vi "qDRL.vi"(0 "System no.":i32=1 min=1 max=4 step=1, 2 "Rec. table to query":i32[](array[numeric]), 3 "With Rec. table IDs?":bool, 5 "error in":errorcluster) -> (16 "No. of rec. values":i32[](array[numeric]), 19 "error out":errorcluster)   [LabVIEW 2020]
doc: "This VI returns the number of recorded data values for the given record tables. \n\nC-887, F-206, M-8X0: Only for GCS syntax version = GCS 2.0 or higher (Check with CSV?.vi. If CSV?.vi is not supported, syntax version is GCS 1.0)."
panel:
  # "Returns the number of recorded data values for the given record tables"
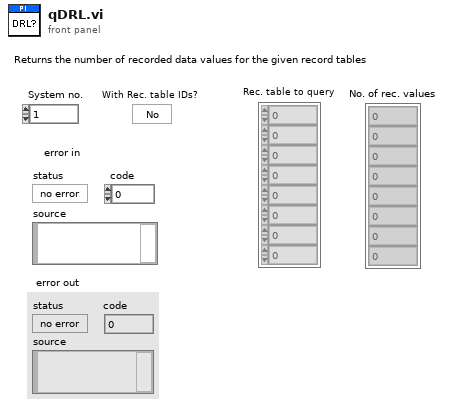
[diagram p1: front panel]
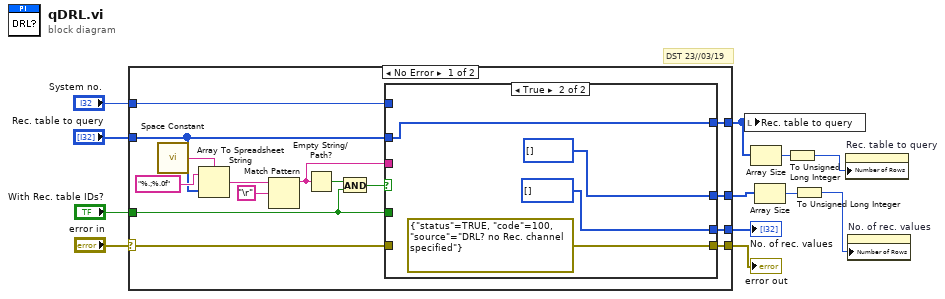
[diagram p0: block diagram]
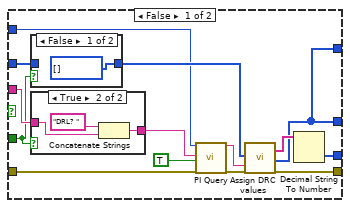
[diagram p2: hidden frame]
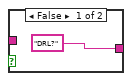
[diagram p4: hidden frame]
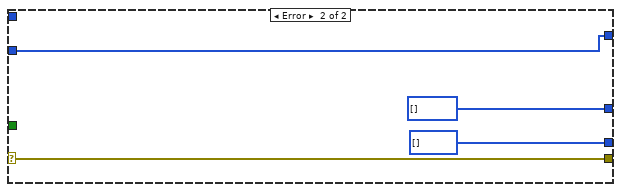
[diagram p5: hidden frame]
diagram:
  # "DST 23//03/19"
  n1 = case shown="No Error" "error in" {
    selector: "error in" -> [w17 w53]
    tunnel: "Rec. table to query" -> [w21 w52]
    tunnel: "System no." -> [w26 _]
    tunnel: [w27 w53] -> w10
    tunnel: "With Rec. table IDs?" -> [w18 _]
    tunnel: [w19 i32[] [] ("Trigger option")] -> w8
    tunnel: [w16 i32[] [] ("Queried Rec. table out")] -> w6
    tunnel: [w13 w52] -> w3
    frame No Error {
      n2 = call <vilib>:"Space Constant.vi"() -> ("String"=w24:string)
      n3 = Array To Spreadsheet String(delimiter (Tab)=w24, array=w21, 3:"%.;%.0f" ("Format String")) -> (spreadsheet string=w22:string)
      n4 = Match Pattern(string=w22, regular expression="\r") -> (before substring=w14:string)  [unwired: 4 out]
      n5 = Empty String/Path?(string/path=w14) -> (empty?=w15:bool)
      n6 = And(x=w15, y=w18) -> (x .and. y?=w20:bool)
      n7 = case shown="True" w20 {
        tunnel: w17 -> [w38 _]
        tunnel: w14 -> [w39 _]
        tunnel: w26 -> [w34 _]
        tunnel: [w37 errorcluster {"status"=TRUE, "code"=100, "source"="DRL? no Rec. channel specified"} ("error out")] -> w27
        tunnel: w21 -> [w36 w48]
        tunnel: [w33 i32[] []] -> w19
        tunnel: w18 -> [w29 _]
        tunnel: [w28 i32[] [] ("Queried Rec. table out")] -> w16
        tunnel: [w28 w48] -> w13
        frame False {
          n8 = case shown="False" w29 {
            tunnel: [i32[] [] ("Rec. table to query") w43] -> w35
            tunnel: w36 -> [_ w43]
            frame False {
            }
            frame True {
            }
          }
          n9 = case shown="True" w29 {
            tunnel: ["DRL?" w46] -> w40
            tunnel: w39 -> [_ w45]
            frame False {
            }
            frame True {
              n10 = Concatenate Strings("DRL? ", w45) -> (w46:string)
            }
          }
          n11 = call "PI Query.vi"("System no."=w34, "String to send"=w40, "Attach termination char.?"=TRUE ("Attach Linefeed?"), "error in"=w38) -> ("String read"=w31:string, "error out"=w30:errorcluster)  [unwired: 3 in, 11 out]
          n12 = call "Assign DRC values.vi"("Queried Rec. table"=w35, "Input String"=w31, "error in"=w30) -> ("Source ID"=w32:string[], "Queried Rec. table out"=w28:i32[], "error out"=w37:errorcluster)  [unwired: 1 in, 13 out]
          n13 = Decimal String To Number(string=w32) -> (number=w33:i32[])  [unwired: 1 in, 2 out]
        }
        frame True {
        }
      }
    }
    frame Error {
    }
  }
  "error out" <- w10
  "No. of rec. values" <- w8
  n14 = local write "Rec. table to query"(w3) -> ()
  n15 = Array Size(array=w3) -> (size(s)=w2:i32)
  n16 = Array Size(array=w6) -> (size(s)=w5:i32)
  n17 = To Unsigned Long Integer(number=w2) -> (unsigned 32bit integer=w1:u32)
  n18 = To Unsigned Long Integer(number=w5) -> (unsigned 32bit integer=w4:u32)
  n19 = property on="Rec. table to query" class="Arr (strict)"("Number of Rows"=w1) -> ()  [unwired: 2 in, 2 out]
  n20 = property on="No. of rec. values" class="Arr (strict)"("Number of Rows"=w4) -> ()  [unwired: 2 in, 2 out]
